vi "Update DDS Arb Buffer.vi"(8 "error in (no error)":errorcluster, 9 "arb_buffer_length":u32, 10 "arb_buffer":u16, 11 "channel_index":u8) -> (0 "error out":errorcluster, 2 "arb_buffer out":u16)   [LabVIEW 2021, in "vmmso.lvlib"]
doc: "DLL_API void WINAPI UpdateDDSArbBuffer(unsigned char channel_index, unsigned short* arb_buffer, unsigned int arb_buffer_length);"
uses:
  vmmso.lvlib
  vmmso.dll
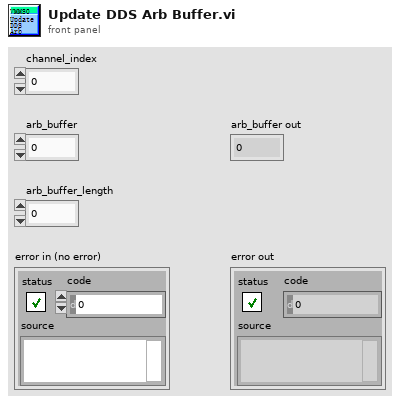
[diagram p1: front panel]
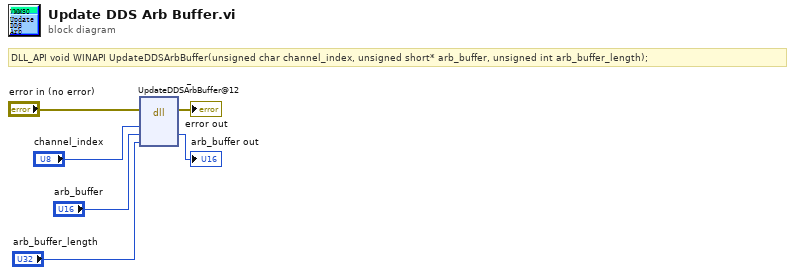
[diagram p0: block diagram]
diagram:
  # "DLL_API void WINAPI UpdateDDSArbBuffer(unsigned char channel_index, unsigned short* arb_buffer, unsigned int arb_buffer_length);"
  n1 = dll-call lib="O:/MSO/library/demo-Labview/vmmso/vmmso.*" fn="_UpdateDDSArbBuffer@12"(error in="error in (no error)", "channel_index"="channel_index", "arb_buffer"="arb_buffer", "arb_buffer_length"="arb_buffer_length") -> (error out=→"error out":errorcluster, "arb_buffer"=→"arb_buffer out":u16)  [unwired: 5 in, 1 out]
